vi "reset.vi"   [LabVIEW 2011]
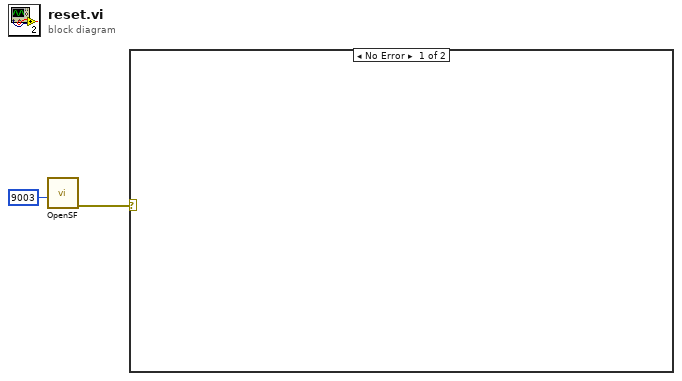
[diagram p0: block diagram]
diagram:
  n1 = call "OpenSF.vi"("port number"=u16 9003) -> ("error out"=w1:errorcluster)  [unwired: 2 out]
  n2 = case shown="No Error" w1 {
    frame No Error {
    }
    frame Error {
    }
  }
